vi "ConvertBrokenDeps10.vi"(1 "dependencies 1.2":T3[](array[typedef]) {"dependee"."component type" items=["standard", "hidden", "system", "unknown", "startup", "image"]; "depender"."component type" items=["standard", "hidden", "system", "unknown", "startup", "image"]}) -> (0 "dependencies 1.0":T1[](array[typedef]))   [LabVIEW 2012]
uses:
  <vilib>/nisyscfg/Broken Dependency 1.2.ctl
  <vilib>/nisyscfg/Software 1.2.ctl
  <vilib>/nisyscfg/Component Type.ctl
  <vilib>/nisyscfg/Broken Dependency.ctl
  <vilib>/nisyscfg/Software.ctl
  <vilib>/nisyscfg/nisyscfg.lvlib
panel:
  # "This cluster is deprecated.\nUse Broken Dependency 1.2.ctl."
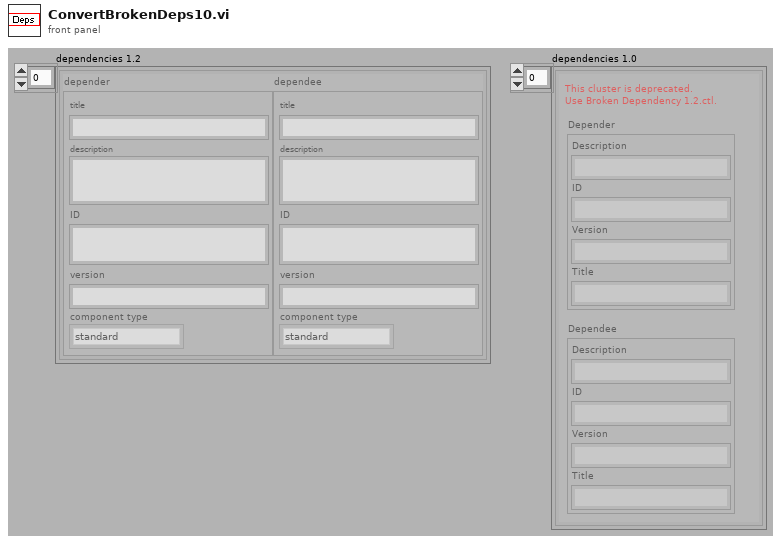
[diagram p1: front panel]
types:
  T1 = typedef "nisyscfg.lvlib/Broken Dependency.ctl" = cluster{"Depender":T2, "Dependee":T2}
  T2 = typedef "nisyscfg.lvlib/Software.ctl" = cluster{"Description":string, "ID":string, "Version":string, "Title":string}
  T3 = typedef "nisyscfg.lvlib/Broken Dependency 1.2.ctl" = cluster{"depender":T4, "dependee":T4}
  T4 = typedef "nisyscfg.lvlib/Software 1.2.ctl" = cluster{"title":string, "description":string, "ID":string, "version":string, "component type":T5}
  T5 = typedef "nisyscfg.lvlib/Component Type.ctl" = u32
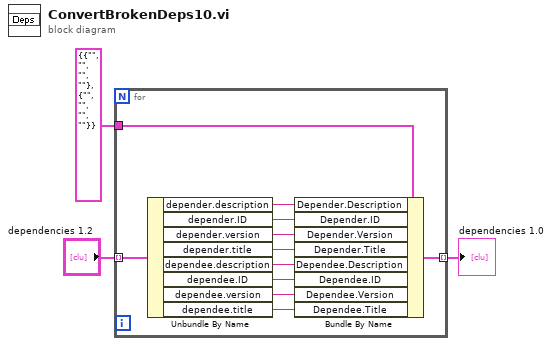
[diagram p0: block diagram]
diagram:
  n1 = for {
    tunnel: T1 {"Depender"={"Description"="", "ID"="", "Version"="", "Title"=""}, "Dependee"={"Description"="", "ID"="", "Version"="", "Title"=""}} ("Broken Dependency") -> [w13]
    tunnel: "dependencies 1.2" -> [w14] mode=indexing
    tunnel: [w12] -> w1 mode=indexing
    n2 = Unbundle By Name(w14) -> ("depender.description"=w11:string, "depender.ID"=w10:string, "depender.version"=w9:string, "depender.title"=w8:string, "dependee.description"=w7:string, "dependee.ID"=w6:string, "dependee.version"=w5:string, "dependee.title"=w4:string)
    n3 = Bundle By Name(cluster=w13, "Depender.Description"=w11, "Depender.ID"=w10, "Depender.Version"=w9, "Depender.Title"=w8, "Dependee.Description"=w7, "Dependee.ID"=w6, "Dependee.Version"=w5, "Dependee.Title"=w4) -> (w12:T1)
  }
  "dependencies 1.0" <- w1
